vi "grapher.vi"() -> ()   [LabVIEW 2016]
panel:
  out "Loops completed":i32
  in  "error in (no error)":errorcluster
  in  "PORT NUMMER":refnum<visa-resource-name>
  out "DATA":cluster{dbl[], dbl[]}(graph)
  in  "Total loops":i32
  out "Voltage":dbl
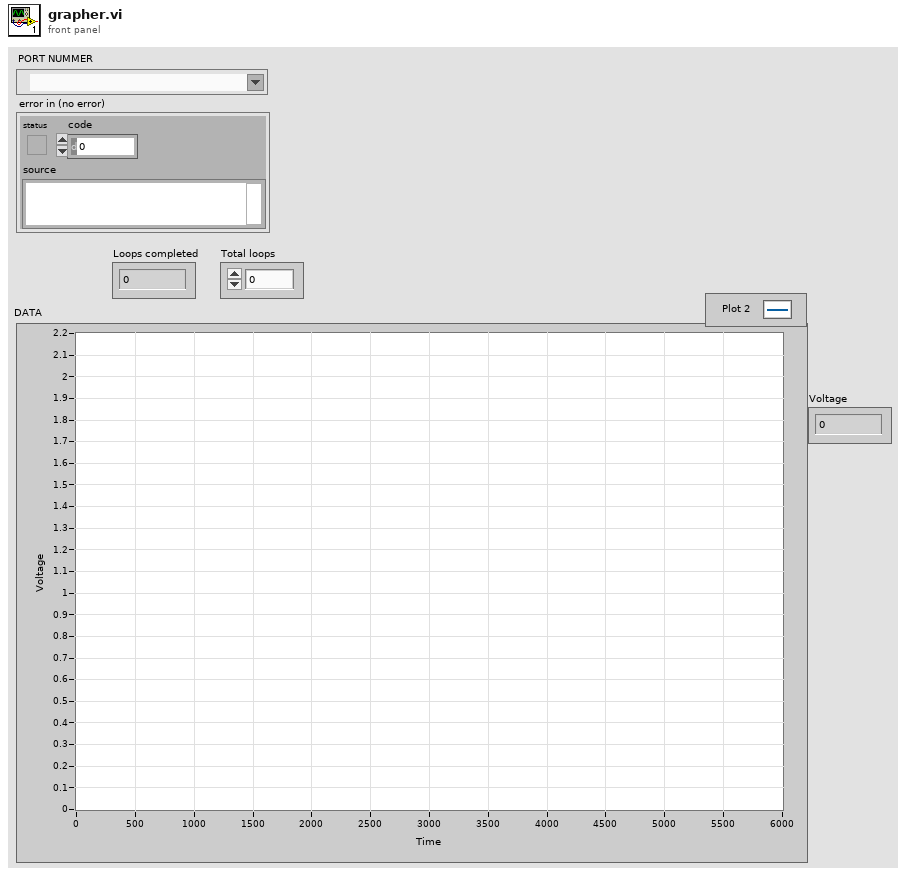
[diagram p1: front panel]
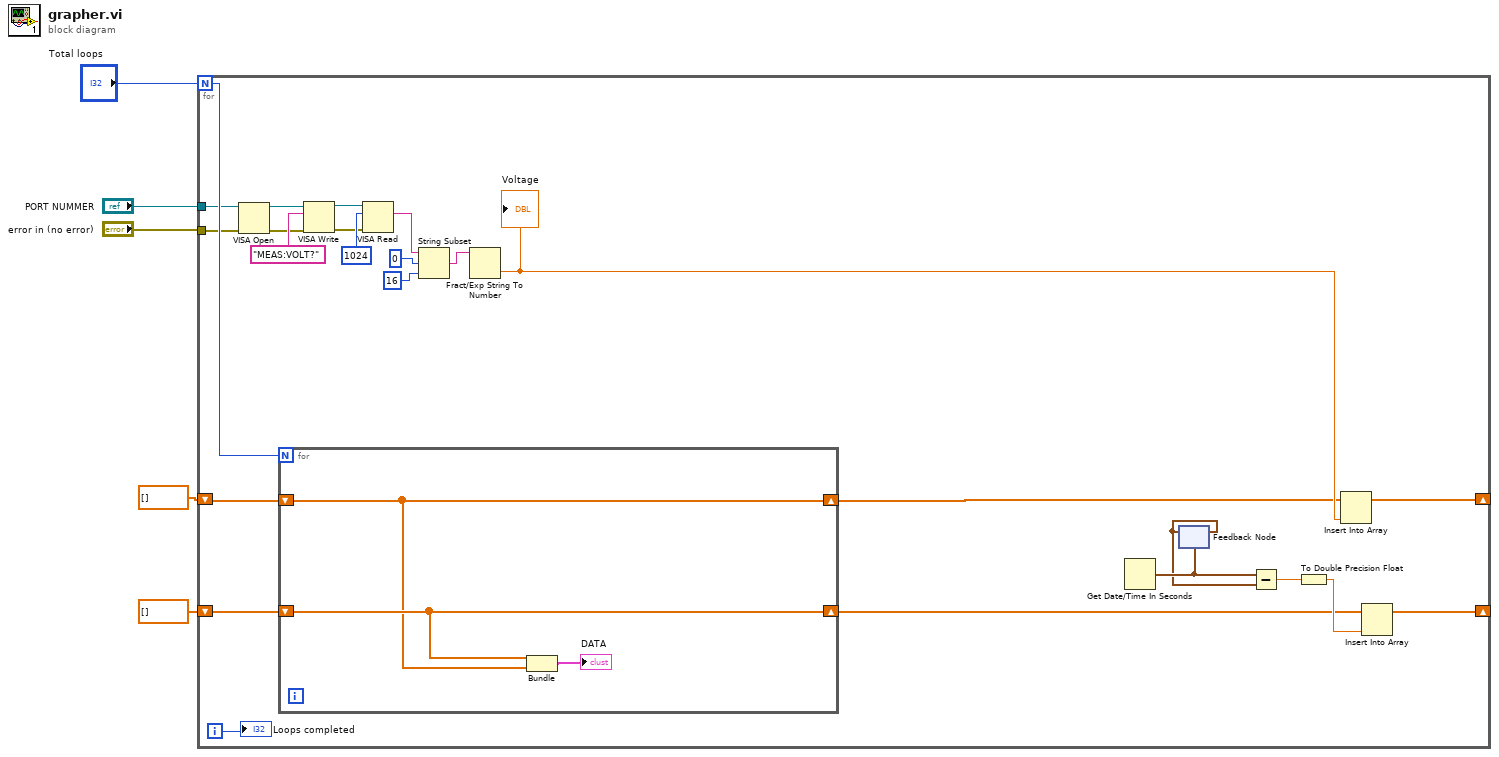
[diagram p0: block diagram]
diagram:
  n1 = for {
    N: "Total loops" -> [w20]
    shift-right: [w17] -> _
    shift-left: dbl[] [] -> [w15]
    shift-right: [w14] -> _
    shift-left: dbl[] [] -> [w13]
    tunnel: "PORT NUMMER" -> [w8]
    tunnel: "error in (no error)" -> [w7]
    i -> [w6]
    n2 = VISA Open(error in (no error)=w7, VISA resource name=w8) -> (VISA resource name=w11:refnum<visa-resource-name>, error out=w10:errorcluster)  [unwired: 3 in]
    n3 = for {
      N: w20 -> [_]
      shift-right: [w32] -> w16
      shift-left: w15 -> [w32]
      shift-right: [w31] -> w12
      shift-left: w13 -> [w31]
      n4 = Bundle(w32, w31) -> (→"DATA":cluster{dbl[], dbl[]})  [unwired: 1 in]
    }
    n5 = VISA Write(VISA resource name=w11, write buffer="MEAS:VOLT?", error in (no error)=w10) -> (VISA resource name out=w27:refnum<visa-resource-name>, error out=w28:errorcluster)  [unwired: 1 out]
    n6 = VISA Read(VISA resource name=w27, byte count=u32 1024, error in (no error)=w28) -> (read buffer=w9:string)  [unwired: 3 out]
    n7 = String Subset(string=w9, offset (0)=0 ("offset"), length (rest)=16 ("offset")) -> (substring=w26:string)
    n8 = Fract/Exp String To Number(string=w26) -> (number=w18:dbl)  [unwired: 3 in, 1 out]
    "Voltage" <- w18
    n9 = Get Date/Time In Seconds() -> (seconds since 1Jan1904=w23:timestamp)
    n10 = feedback #1(w23) -> (w22:timestamp)
    n11 = feedback-in #1(w22) -> ()
    n12 = Subtract(x=w23, y=w22) -> (x-y=w21:dbl)
    n13 = To Double Precision Float(number=w21) -> (double precision float=w19:dbl)
    n14 = Insert Into Array(array=w12, new element=w18) -> (w14:dbl[])  [unwired: 1 in]
    n15 = Insert Into Array(array=w16, new element=w19) -> (w17:dbl[])  [unwired: 1 in]
    "Loops completed" <- w6
  }
